vi "AboutGui.vi"() -> ()   [LabVIEW 2016]
uses:
  Global/ApplicationGlobal.vi
panel:
  out "Changelog":string caption="MAKE CURRENT VALUE DEFAULT!!!"
  in  "OKButton":bool
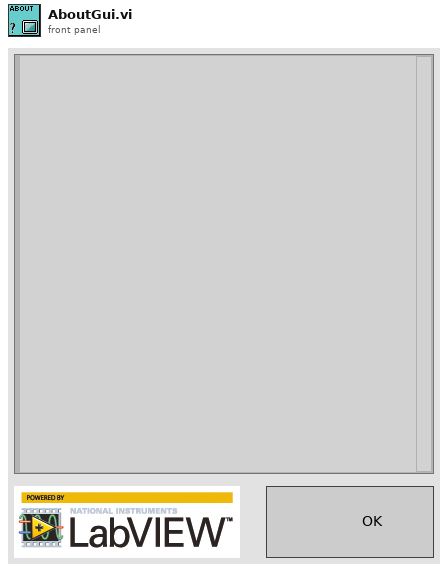
[diagram p1: front panel]
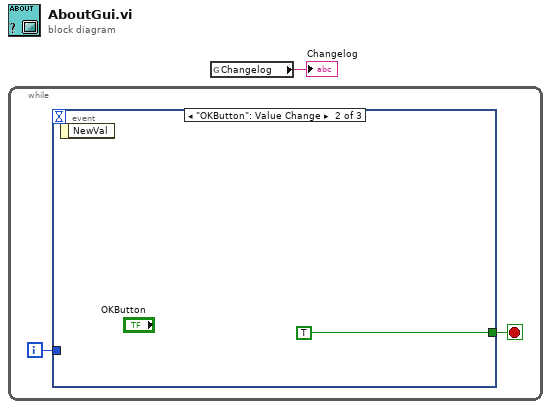
[diagram p0: block diagram]
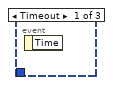
[diagram p2: hidden frame]
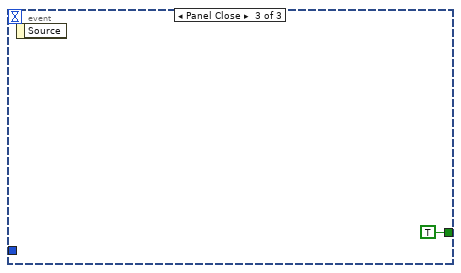
[diagram p3: hidden frame]
diagram:
  n1 = while "Respond to User" {
    i -> [w2]
    stop <- w3 stop-if-true
    n2 = event shown="[1] \"OKButton\": Value Change" {
      selector: _ -> [_ _ _]
      dyn-events: _ -> [_ _ _]
      timeout: _ -> [_ _ _]
      tunnel: [_ TRUE TRUE] -> w3
      tunnel: w2 -> [_ _ _]
      event Timeout {
        n3 = event-data() -> ()  [unwired: 2 out]
      }
      event "OKButton": Value Change {
        n4 = event-data() -> ()  [unwired: 2 out]
      }
      event Panel Close {
        n5 = event-data() -> ()  [unwired: 2 out]
      }
    }
  }
  n6 = global read "ApplicationGlobal.vi" "Changelog"() -> (→"Changelog":string)
